vi "Read 433x.vi"(5 "Late?":bool, 8 "error in (no error)":errorcluster, 11 "433x in":T1) -> (0 "error out":errorcluster, 3 "433x out":T1)   [LabVIEW 2011, in "PXIe-433x Custom Device.lvlib"]
uses:
  PXIe-433x Custom Device.lvlib
  433x data.ctl
  <vilib>/DAQmx/read.llb/DAQmx Read.vi
  <vilib>/DAQmx/read.llb/DAQmx Read (Analog 2D DBL NChan NSamp).vi
  <vilib>/DAQmx/miscellaneous.llb/DAQmx Fill In Error Info.vi
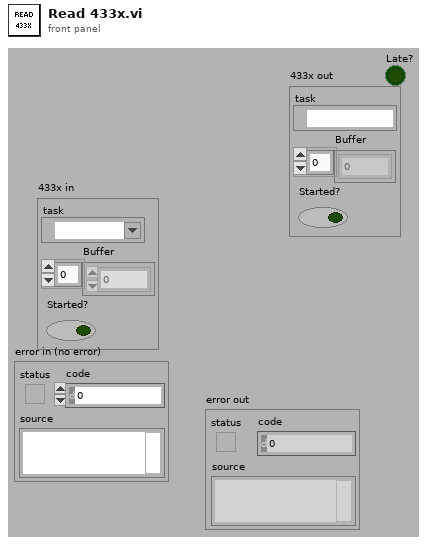
[diagram p1: front panel]
types:
  T1 = typedef "PXIe-433x Custom Device.lvlib/433x data.ctl" = cluster{"task":refnum<k21>, "Buffer":dbl[], "Started?":bool}
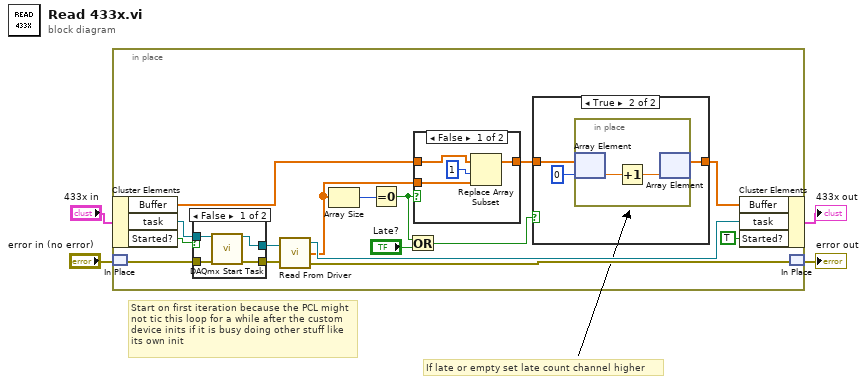
[diagram p0: block diagram]
diagram:
  # "Start on first iteration because the PCL might not tic this loop for a while after the custom device inits if it is busy doing other stuff like its own init"
  # "If late or empty set late count channel higher"
  n1 = in-place {
    n2 = in-place-cluster #1("433x in") -> ("Buffer"=w15:dbl[], "task"=w8:refnum<k21>, "Started?"=w6:bool)
    n3 = in-place-match #2("error in (no error)") -> (w13:errorcluster)
    n4 = case shown="False" w6 {
      tunnel: w13 -> [w24 w25]
      tunnel: [w23 w25] -> w9
      tunnel: w8 -> [w22 w26]
      tunnel: [w21 w26] -> w7
      frame False {
        n5 = call <vilib>:"DAQmx Start Task.vi"("task/channels in"=w22, "error in"=w24) -> ("task out"=w21:refnum<k21>, "error out"=w23:errorcluster)  [unwired: 12 in]
      }
      frame True {
      }
    }
    n6 = call "Read From Driver.vi"("error in"=w9, "task in"=w7) -> ("error out"=w11:errorcluster, "data"=w10:dbl[], "task out"=w12:refnum<k21>)
    n7 = Array Size(array=w10) -> (size(s)=w20:i32)
    n8 = Equal To 0?(x=w20) -> (x = 0?=w16:bool)
    n9 = Or(x=w16, y="Late?") -> (x .or. y?=w17:bool)
    n10 = case shown="False" w16 {
      tunnel: w15 -> [w30 w31]
      tunnel: w10 -> [w28 _]
      tunnel: [w27 w31] -> w14
      frame False {
        n11 = Replace Array Subset(array=w30, new element=w28, index=1) -> (w27:dbl[])
      }
      frame True {
      }
    }
    n12 = case shown="True" w17 {
      tunnel: w14 -> [w32 w35]
      tunnel: [w32 w34] -> w19
      frame False {
      }
      frame True {
        n13 = in-place {
          n14 = in-place-array #3(w35, 0) -> (w37:dbl)
          n15 = Increment(x=w37) -> (x+1=w36:dbl)
          n16 = in-place-array #3(w36) -> (w34:dbl[])  [unwired: 1 out]
        }
      }
    }
    n17 = in-place-cluster #1("Buffer"=w19, "task"=w12, "Started?"=TRUE) -> (→"433x out":T1)
    n18 = in-place-match #2(w11) -> (→"error out":errorcluster)
  }
